vi "Close.vi"(8 "error in (no error)":errorcluster, 11 "Tektronix DMM4020 in":refnum<class "Tektronix DMM4020.lvclass">) -> (0 "error out":errorcluster, 3 "Tektronix DMM4020 out":refnum<class "Tektronix DMM4020.lvclass">)   [LabVIEW 2014, in "Generic Digital Multi Meter.lvlib" / "Tektronix DMM4020.lvlib" / "Tektronix DMM4020.lvclass"]
uses:
  Tektronix DMM4020.lvclass
  <instrlib>/Tektronix DMM4020/Tektronix DMM4020.lvlib
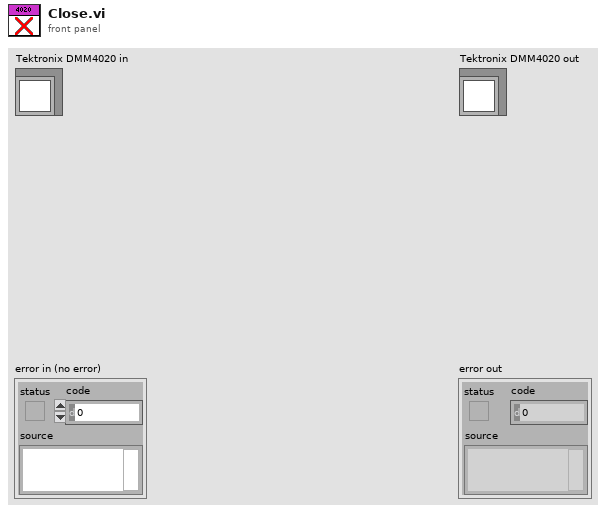
[diagram p1: front panel]
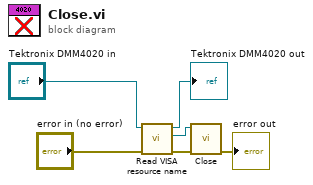
[diagram p0: block diagram]
diagram:
  n1 = call-dynamic "Read VISA resource name.vi"("error in (no error)"="error in (no error)", "Generic Instrument in"="Tektronix DMM4020 in") -> ("error out"=w4:errorcluster, "VISA resource name"=w5:refnum<visa-resource-name>, "Generic Instrument out"=→"Tektronix DMM4020 out":refnum<class "Tektronix DMM4020.lvclass">)  [unwired: 7 in]
  n2 = call <instrlib>:"Close.vi"("error in (no error)"=w4, "VISA resource name"=w5) -> ("error out"=→"error out":errorcluster)  [unwired: 9 in]
